vi "信号光谱5.vi"() -> ()   [LabVIEW 2018]
uses:
  <vilib>/Instr/_visa.llb/VISA Configure Serial Port (Instr).vi
  <vilib>/Utility/file.llb/Write Delimited Spreadsheet (DBL).vi
  <vilib>/Analysis/NI_AALBase.lvlib
  <vilib>/ptbypt/NI_PtbyPt.lvlib
panel:
  in  "阈值条件":dbl
  in  "判断角度":dbl
  in  "input parameter":string="D:\\1.jpg"
  out "error out 3":errorcluster
  out "error out 2":errorcluster
  out "照明光":bool
  in  "stop bits (10: 1 bit)":u16(ring)=10 items=["1.0"=10, "1.5"=15, "2.0"=20]
  in  "parity (0:none)":enum16{"None", "Odd", "Even", "Mark", "Space"}(ring)
  in  "data bits (8)":u16=8 min=5 max=8 step=1
  in  "baud rate":u32=9600 caption="baud rate (115200)" min=9600 max=115200
  in  "VISA resource name":refnum<visa-resource-name>="COM3"
  out "正在测量":bool
  in  "滤波阈值":dbl=1500.0 format="%#_13g"
  out "best fit":dbl[][](graph) caption="最佳拟合"
  out "范围内？":bool[](array[boolean])
  out "w":dbl
  out "xc":dbl
  out "拟合参数":dbl[](array[numeric])
  out "最终存储路径":path
  in  "停止程序":bool
  in  "上升下降沿/s":dbl format="%.2p"
  in  "延时/s":dbl format="%.2p"
  in  "占空比/%":dbl=3.0 format="%.2p"
  in  "高电平/V":dbl=4.0 format="%.2p"
  in  "频率/Hz":dbl=100.0 format="%.3p"
  in  "低电平/V":dbl min=0.0 max=5.0 format="%.2p"
  out "configure error out":errorcluster
  in  "设置参数":bool
  out "output control error  4":errorcluster
  in  "低电平持续输出":bool
  in  "Output 1":bool
  out "output control error  5":errorcluster
  in  "测量高电平/V":dbl=4.0
  out "output control error  2":errorcluster
  in  "开始测量":bool
  in  "上升下降沿":i32(ring)=1 items=["上升沿", "下降沿"]
  in  "channel输出口":i32(ring) items=["Channel 1", "Channel 2"]
  in  "输出信号波形":u16(ring) items=["Pulse"]
  out "output control error  3":errorcluster
  out "Output":bool
  in  "VISA 信号发生器":refnum<visa-resource-name>="USB0::0x1AB1::0x0641::DG4E192200870::INSTR"
  out "Spectrum":cluster{"Y":dbl[], "Y":dbl[]}[](graph)
  in  "计数器":dbl=720.0
  out "波长范围":dbl[](array[numeric])
  in  "选项卡控件":enum32{"IHR 550", "CCD"}(tab)
  in  "Move To\nTarget Positions":bool
  out "Current UniqueID":string="Mono4"
  in  "Mono ID":string(combo)="Mono1"
  in  "Connect":bool
  out "Initialized JY":bool=TRUE
  in  "Force\nInitialization":bool
  in  "Target Grating":string(combo)="2"
  out "Current Description":string="1" caption="Description"
  out "Grating Index":i32=1
  out "Current Grating":dbl=1200.0
  out "Units":string="nm"
  out "Current WL":dbl=897.9988
  out "Exit Mirror\nPosition":i32(ring)=2 items=["EntranceMirror", "ExitMirror", "Front", "Side"]
  out "Entrance Mirror\nPosition":i32(ring)=2 items=["EntranceMirror", "ExitMirror", "Front", "Side"]
  out "Units 2":string="mm"
  out "Front Entrance":dbl
  in  "Target WL":dbl=2670.0
  in  "Exit Mirror":u16(ring)=3 caption="Target Position Exit Mirror" items=["Front"=2, "Side"=3]
  in  "Entrance Mirror":u16(ring)=2 caption="Target Position\nEntrance Mirror" items=["Front"=2, "Side"=3]
  in  "Target\nFront Entrance":dbl=1.0
  in  "Commande tab":T1(tab)
  in  "Area Number to Display":i32
  in  "Reformat":bool
  in  "GAIN":u16(ring)=2 caption="Device Name" items=["High Light", "Best Dynamic Range", "High Sensitivity"]
  in  "ADC":u16(ring) caption="Device Name" items=["20 kHz       ", " 1 MHz       ", " 1 MHz Ultra "]
  in  "Number of Areas :":u16=1 min=1 step=1
  in  "Integration time (ms) :":i16=5000
  out "Uniques ID":u16(ring) items=["CCD1", "CCD2"]
  in  "Device Name":u16(ring) items=["Synapse CCD (Lateral)", "Synapse_IGA (Axial)"]
  in  "Signal type :":enum16{"TTL Rising Edge", "TTL Falling Edge"}(ring)=enum."TTL Falling Edge"
  in  "Trigger Type :":u16(ring) items=["On Start"=1, "Per Acquisition"=2]
  in  "trigSigTypeString":string
  in  "trigEventString":string
  in  "Enable InputTriggers :":bool
  in  "Number of Cleans":i32=1
  in  "MultiAcqShutterMode":i32(ring)=3 items=["Open For All Spectra"=1, "Open for Each Spectrum"=3]
  in  "Accumulations:":u16=10 min=1 step=1
  in  "Multi Accumulation mode:":bool
  out "Y Pixels:":i32=256
  out "DataSize":i32=1024
  out "X Pixels:":i32=1024
  out "Firmware\nVersion":string="V1.20 CCD_4000"
  out "initialized ?":bool=TRUE
  in  "Continuous":bool
  in  "CCD Busy":bool
  out "indicator":string="Ready !"
  in  "initialize":bool
  in  "ShutterOpen":bool=TRUE caption="Shutter enable"
  in  "Acquire":bool
  in  "Temperature":bool
  in  "Setup":bool
  in  "起始波长":dbl=2406.79
  in  "终止波长":dbl=2919.91
  out "Acq Time(ms)":u32=3401
  in  "Save Backlight":bool
  in  "cut backlight":bool
  out "backlight":bool=TRUE
  in  "Close":bool=TRUE
  out "JYCCDLib.IJYCCDReqd":refnum<k7>
  out "areas :":i32[][](array[numeric])=[[1], [1], [1], [1024], [256], [1], [256]]
  in  "Constante de condition\n(Voir l'aide contextuelle)":bool
  out "temp graph":dbl(graph)=-134.538067
  out "ADC Number":i32[](array[numeric])=[0, 1, 2, 3, 4]
  out "Gain Number":i32[](array[numeric])=[10, 11, 12, 13, 8, 2]
  out "trigAddress":i32
  out "Data":i32[][](graph)
  out "error out":errorcluster
  out "Gratings":dbl[](array[numeric])=[1200.0, 300.0]
  out "Backlight":i32[][](graph)
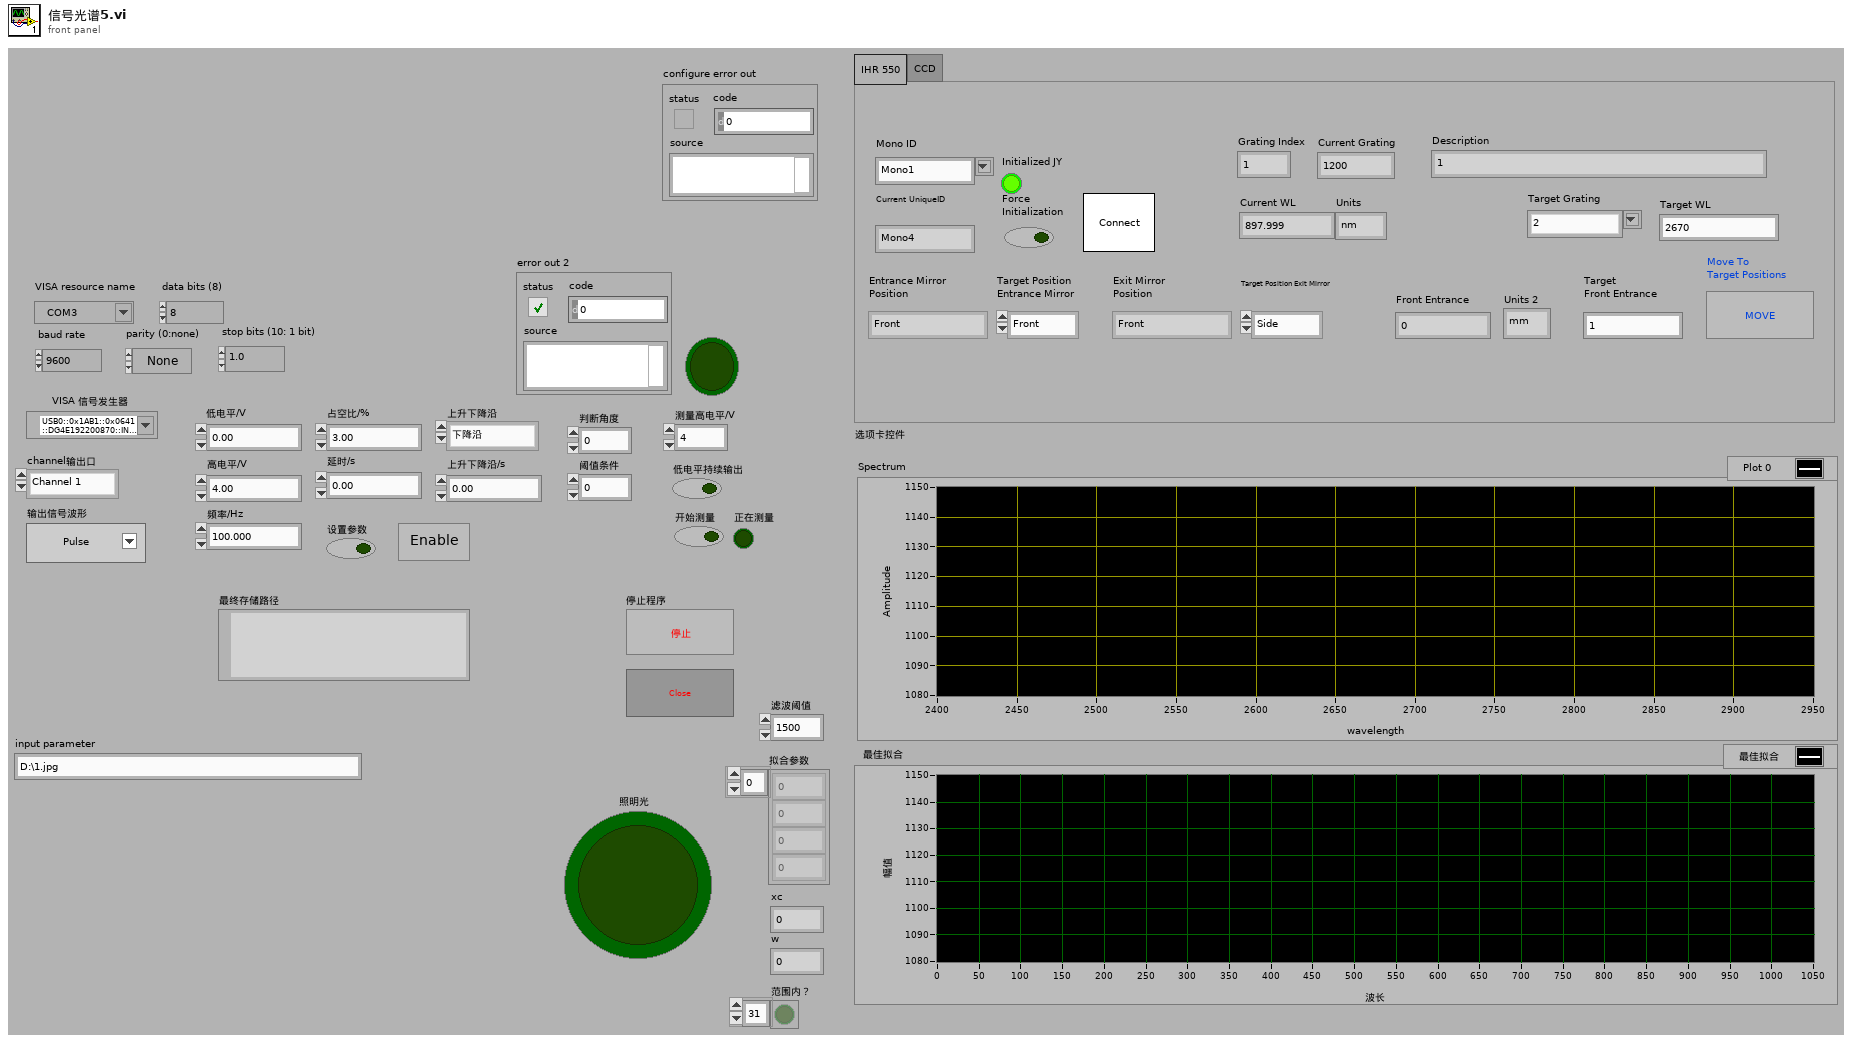
[diagram p1: front panel]
types:
  T1 = enum32{"Settings", "Trigger In", "Multi-Accu.", "Infos"}
  T2 = enum8{"Enabled", "Disabled", "Disabled and Grayed Out"}
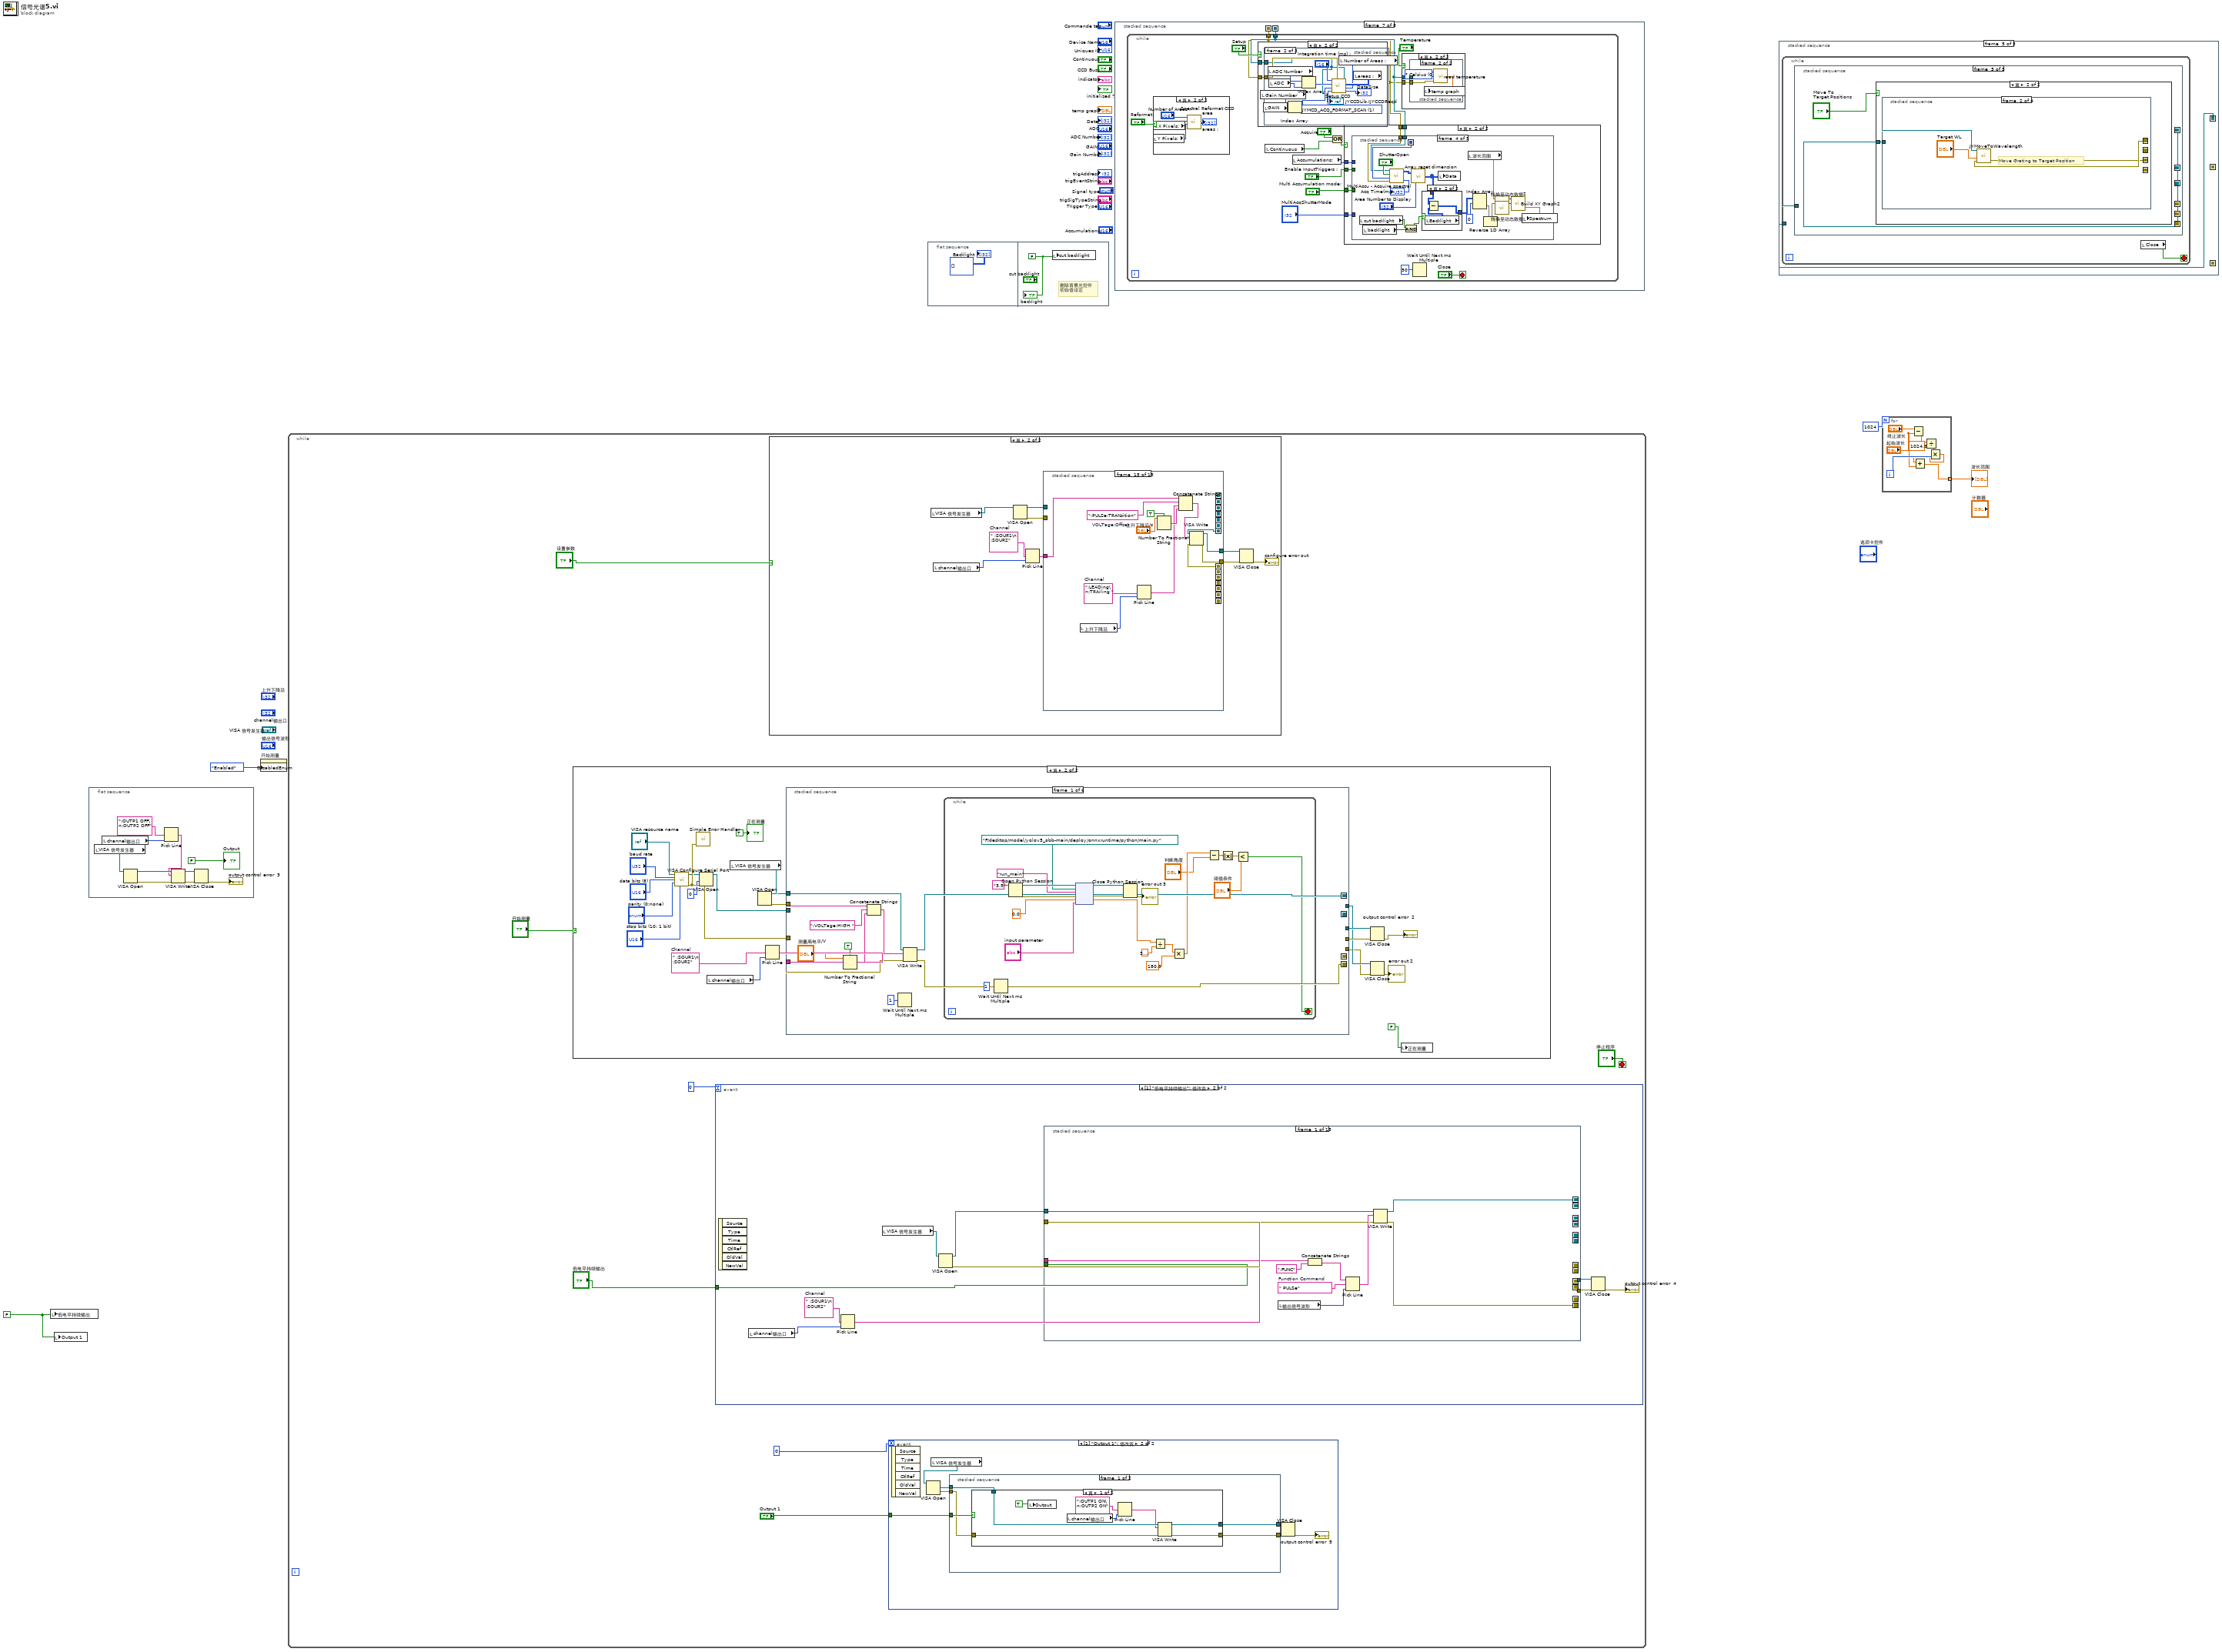
[diagram p0: block diagram]
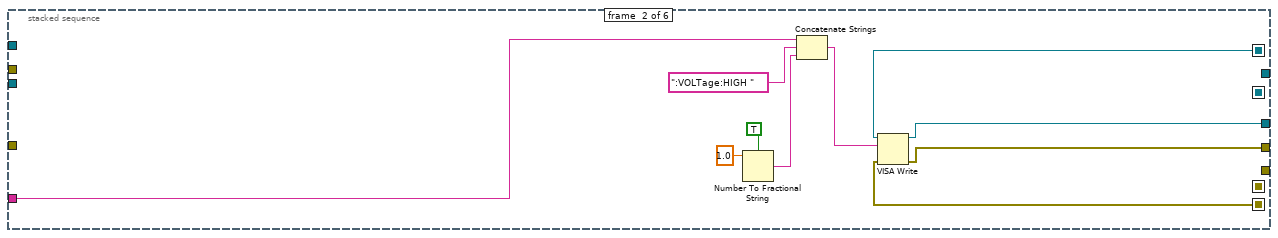
[diagram p3: hidden frame]
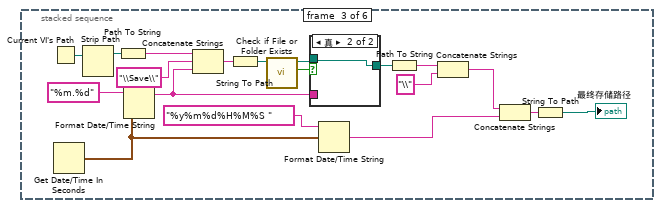
[diagram p4: hidden frame]
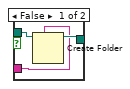
[diagram p5: hidden frame]
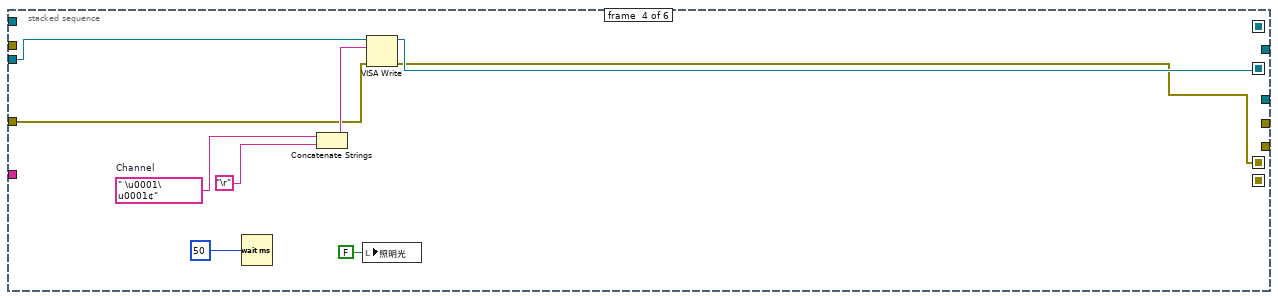
[diagram p6: hidden frame]
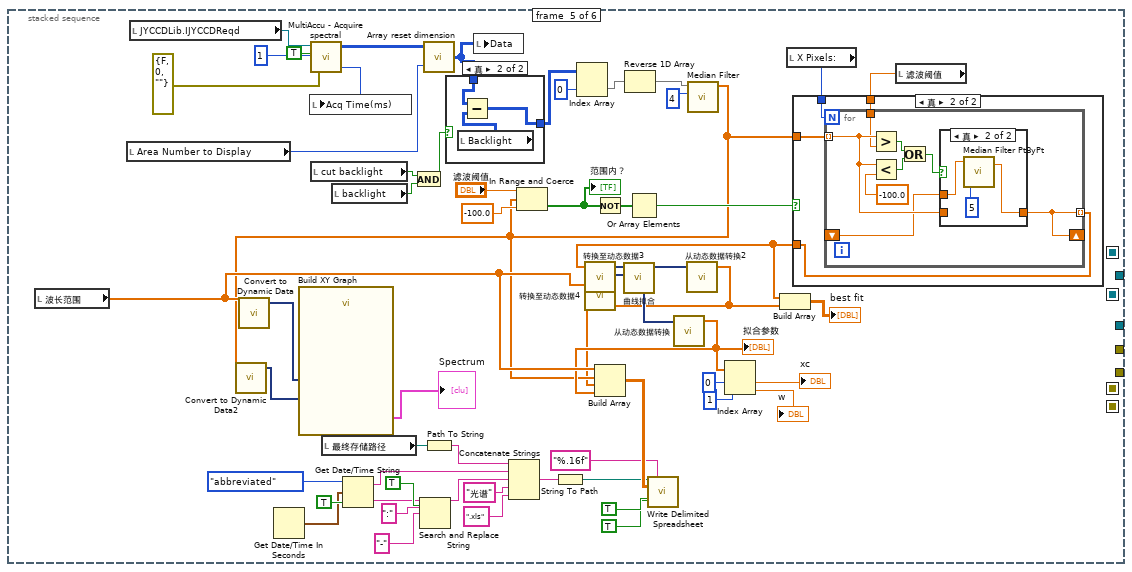
[diagram p7: hidden frame]
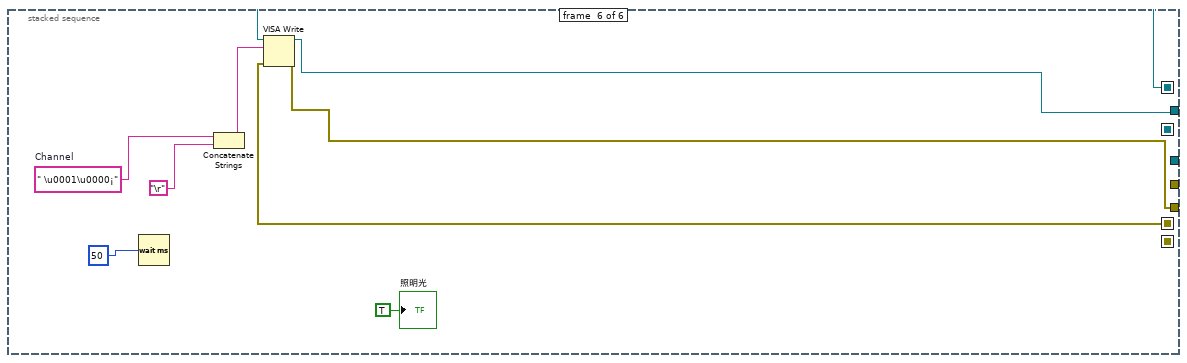
[diagram p11: hidden frame]
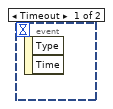
[diagram p12: hidden frame]
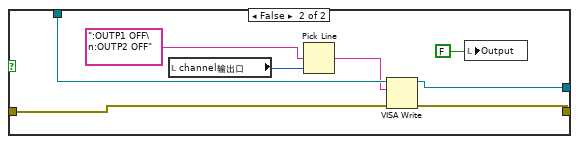
[diagram p13: hidden frame]
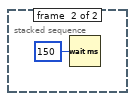
[diagram p14: hidden frame]
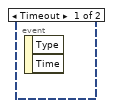
[diagram p15: hidden frame]
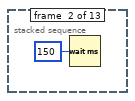
[diagram p16: hidden frame]
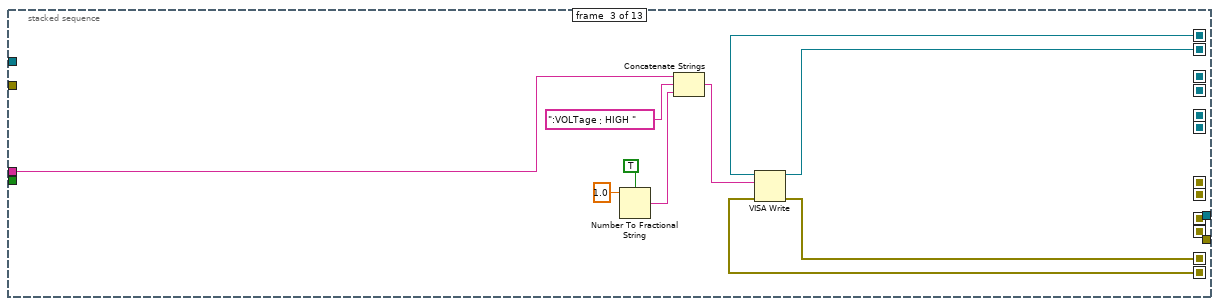
[diagram p17: hidden frame]
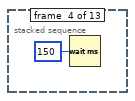
[diagram p18: hidden frame]
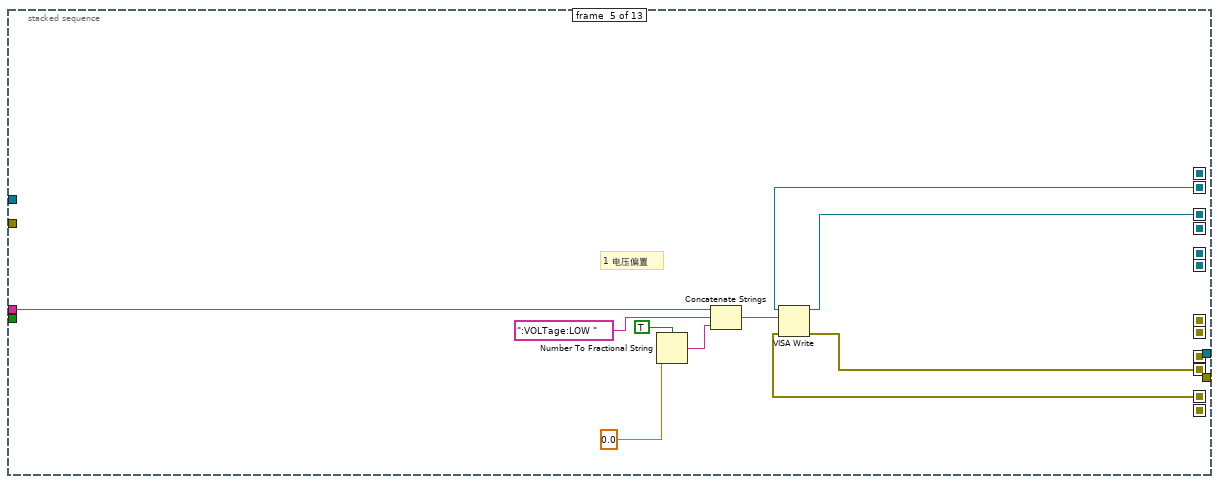
[diagram p19: hidden frame]
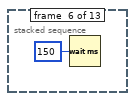
[diagram p20: hidden frame]
diagram:
  w1 = FALSE
  n1 = local write "低电平持续输出"(w1) -> ()
  n2 = local write "Output 1"(w1) -> ()
  n3 = flat-sequence {
    frame #0 {
      n4 = local read "VISA 信号发生器"() -> (w8:refnum<visa-resource-name>)
      n5 = local read "channel输出口"() -> (w6:i32)
      n6 = VISA Open(VISA resource name=w8) -> (VISA resource name=w14:refnum<visa-resource-name>, error out=w13:errorcluster)  [unwired: 4 in]
      n7 = Pick Line(multi-line string=":OUTP1 OFF\n:OUTP2 OFF" ("write buffer"), line index=w6) -> (output string=w5:string)  [unwired: 1 in]
      n8 = VISA Write(VISA resource name=w14, write buffer=w5, error in (no error)=w13) -> (VISA resource name out=w11:refnum<visa-resource-name>, error out=w10:errorcluster)  [unwired: 1 out]
      n9 = VISA Close(VISA resource name=w11, error in (no error)=w10) -> (error out=→"output control error  3":errorcluster)
      "Output" <- FALSE ("布尔")
    }
  }
  n10 = property on="开始测量" class="Bool"("DisabledEnum"=T2."Enabled" ("禁用")) -> ()  [unwired: 2 in, 2 out]
  n11 = while {
    stop <- "停止程序" stop-if-true
    n12 = case shown="真" "开始测量" {
      frame False {
      }
      frame True {
        w37 = " :SOUR1\n :SOUR2"  # Channel
        n13 = call-poly "VISA Configure Serial Port"("VISA resource name"="VISA resource name", "baud rate (9600)"="baud rate", "data bits (8)"="data bits (8)", "parity (0:none)"="parity (0:none)", "stop bits (10: 1 bit)"="stop bits (10: 1 bit)") -> ("VISA resource name out"=w30:refnum<visa-resource-name>, "error out"=w31:errorcluster)  [unwired: 9 in]
        n14 = call <vilib>:"Simple Error Handler.vi"("error in (no error)"=w31) -> ()  [unwired: 4 in, 5 out]
        n15 = VISA Open(access mode=0, error in (no error)=w31, VISA resource name=w30) -> (VISA resource name=w23:refnum<visa-resource-name>, error out=w22:errorcluster)  [unwired: 2 in]
        n16 = local read "channel输出口"() -> (w38:i32)
        n17 = local read "VISA 信号发生器"() -> (w44:refnum<visa-resource-name>)
        n18 = VISA Open(VISA resource name=w44) -> (VISA resource name=w43:refnum<visa-resource-name>, error out=w42:errorcluster)  [unwired: 4 in]
        n19 = Pick Line(multi-line string=w37, line index=w38) -> (output string=w36:string)  [unwired: 1 in]
        n20 = stacked-sequence {
          seq-local: [w48 _ _ _ _ _] -> [_ w80 _ _ _ w202]
          seq-local: [w47 _ _ _ _ _] -> [_ w79 _ _ _ _]
          seq-local: [_ _ _ w112 _ _] -> [_ _ _ _ _ _]
          seq-local: [_ _ _ w111 _ _] -> [_ _ _ _ _ w203]
          tunnel: w43 -> [w51 _ _ _ _ _]
          tunnel: w42 -> [w50 _ _ _ _ _]
          tunnel: [_ w82 _ _ _ _] -> w41
          tunnel: [_ w81 _ _ _ _] -> w40
          tunnel: w36 -> [w52 w78 _ _ _ _]
          tunnel: w23 -> [_ _ _ w115 _ _]
          tunnel: w22 -> [_ _ _ w114 _ _]
          tunnel: [_ _ _ _ _ w201] -> w34
          tunnel: [_ _ _ _ _ w200] -> w33
          frame #0 {
            n21 = Number To Fractional String(use system decimal point (T)=TRUE ("使用系统小数点(T)"), number="测量高电平/V") -> (F-format string=w54:string)  [unwired: 2 in]
            n22 = Concatenate Strings ("连接字符串")(w52, ":VOLTage:HIGH ", w54) -> (w53:string)
            n23 = Wait Until Next ms Multiple(millisecond multiple=u32 1 ("毫秒倍数")) -> ()  [unwired: 1 out]
            n24 = VISA Write(VISA resource name=w51, write buffer=w53, error in (no error)=w50) -> (VISA resource name out=w48:refnum<visa-resource-name>, error out=w47:errorcluster)  [unwired: 1 out]
            n25 = while {
              stop <- w59 stop-if-true
              n26 = Wait Until Next ms Multiple(millisecond multiple=u32 1 ("毫秒倍数")) -> ()  [unwired: 1 out]
              n27 = Open Python Session(python version="3.9" ("Python version")) -> (session out=w76:refnum<k35>, error out=w74:errorcluster)  [unwired: 2 in]
              n28 = node(w76, path "F:/desktop/model/yolov5_obb-main/deploy/onnxruntime/python/main.py" ("module path"), "run_main" ("function name"), w74, 0.0, "input parameter") -> (w75:refnum<k35>, w73:errorcluster, w57:dbl)  [unwired: 1 in, 2 out]
              n29 = Close Python Session(session in=w75, error in=w73) -> (11:→"error out 3":errorcluster)
              n30 = Divide(x=w57, y=3.141592653589793) -> (x/y=w66:dbl)
              n31 = Multiply(x=w66, y=180.0) -> (x*y=w64:dbl)
              n32 = Subtract(x=w64, y="判断角度") -> (x-y=w62:dbl)
              n33 = Absolute Value(x=w62) -> (abs(x)=w61:dbl)
              n34 = Less?(x=w61, y="阈值条件") -> (x < y?=w59:bool)
            }
          }
          frame #1 {
            n35 = Number To Fractional String(use system decimal point (T)=TRUE ("使用系统小数点(T)"), number=1.0 ("数字")) -> (F-format string=w85:string)  [unwired: 2 in]
            n36 = Concatenate Strings ("连接字符串")(w78, ":VOLTage:HIGH ", w85) -> (w84:string)
            n37 = VISA Write(VISA resource name=w80, write buffer=w84, error in (no error)=w79) -> (VISA resource name out=w82:refnum<visa-resource-name>, error out=w81:errorcluster)  [unwired: 1 out]
          }
          frame #2 {
            n38 = Current VI's Path() -> (path=w93:path)
            n39 = Get Date/Time In Seconds() -> (seconds since 1Jan1904=w95:timestamp)
            n40 = Strip Path(path=w93) -> (stripped path=w94:path)  [unwired: 1 out]
            n41 = Path To String(path=w94) -> (string=w96:string)
            n42 = Format Date/Time String(time format string (%c)="%m.%d" ("时间格式字符串(%c)"), seconds (now)=w95) -> (date/time string=w102:string)  [unwired: 1 in]
            n43 = Concatenate Strings(w96, "\\Save\\" ("字符串"), w102) -> (w97:string)
            n44 = String To Path(string=w97) -> (path=w98:path)
            n45 = call <vilib>:"Check if File or Folder Exists.vi"("path"=w98) -> ("file or folder exists?"=w99:bool, "dup path"=w101:path)  [unwired: 8 in, 1 out]
            n46 = case shown="真" w99 {
              tunnel: [w109 w110] -> w100
              tunnel: w101 -> [w108 w110]
              tunnel: w102 -> [w107 _]
              frame False {
                n47 = Create Folder(prompt (Create Folder)=w107, path (use dialog)=w108) -> (created path=w109:path)  [unwired: 1 in, 2 out]
              }
              frame True {
              }
            }
            n48 = Format Date/Time String(time format string (%c)="%y%m%d%H%M%S " ("时间格式字符串(%c)"), seconds (now)=w95) -> (date/time string=w105:string)  [unwired: 1 in]
            n49 = Path To String(path=w100) -> (string=w103:string)
            n50 = Concatenate Strings(w103, "\\" ("字符串")) -> (w104:string)
            n51 = Concatenate Strings(w104, w105) -> (w92:string)
            n52 = String To Path(string=w92) -> (path=→"最终存储路径":path)
          }
          frame #3 {
            w116 = " \u0001\u0001¢"  # Channel
            n53 = Wait (ms)(milliseconds to wait=50) -> ()  [unwired: 1 out]
            n54 = Concatenate Strings(w116, "\r") -> (w117:string)
            n55 = local write "照明光"(FALSE ("照明光")) -> ()
            n56 = VISA Write(VISA resource name=w115, write buffer=w117, error in (no error)=w114) -> (VISA resource name out=w112:refnum<visa-resource-name>, error out=w111:errorcluster)  [unwired: 1 out]
          }
          frame #4 {
            n57 = local read "波长范围"() -> (w142:dbl[])
            n58 = local read "Area Number to Display"() -> (w152:i32)
            n59 = local read "JYCCDLib.IJYCCDReqd"() -> (w148:refnum<k7>)
            n60 = call "Convert to Dynamic Data"("Array"=w142) -> ("Dynamic Data Type"=w145:dynamicdata)  [unwired: 3 in]
            n61 = Get Date/Time In Seconds() -> (seconds since 1Jan1904=w161:timestamp)
            n62 = call "MultiAccu - Acquire spectral.vi"("error in"=errorcluster {"status"=FALSE, "code"=0, "source"=""}, "Accumulations:"=u16 1, "ShutterOpen"=TRUE, "JYCCDLib.IJYCCDReqd"=w148) -> ("Acq Time(ms)"=w154:u32, "Array Out"=w153:i32[][][])  [unwired: 1 out]
            n63 = local write "Acq Time(ms)"(w154) -> ()
            n64 = local read "cut backlight"() -> (w133:bool)
            n65 = local read "最终存储路径"() -> (w175:path)
            n66 = local read "backlight"() -> (w131:bool)
            n67 = Get Date/Time String(date format (0)=enum16{"short", "long", "abbreviated"}."abbreviated" ("日期格式(0)"), seconds (now)=w161, want seconds? (F)=TRUE ("需要秒？(F)")) -> (date string=w169:string, time string=w164:string)
            n68 = And(x=w133, y=w131) -> (x .and. y?=w132:bool)
            n69 = Search and Replace String(replace all?=TRUE ("替换全部？(F)"), input string=w164, search string=":" ("搜索字符串"), replace string="-" ("替换字符串(\"\")")) -> (result string=w168:string)  [unwired: 4 in, 3 out]
            n70 = call "Array reset dimension.vi"("Area Number"=w152, "Array In"=w153) -> ("Array Out"=w135:i32[][])
            n71 = Path To String(path=w175) -> (string=w158:string)
            n72 = case shown="真" w132 {
              tunnel: [w196 w198] -> w134
              tunnel: w135 -> [w196 w197]
              frame False {
              }
              frame True {
                n73 = local read "Backlight"() -> (w199:i32[][])
                n74 = Subtract(x=w197, y=w199) -> (x-y=w198:i32[][])
              }
            }
            n75 = local write "Data"(w135) -> ()
            n76 = Concatenate Strings(w158, w169, w168, "光谱" ("字符串"), ".xls" ("字符串")) -> (w173:string)
            n77 = String To Path(string=w173) -> (path=w174:path)
            n78 = Index Array(array=w134, index (row)=0 ("索引 (行)")) -> (element=w176:i32[])  [unwired: 1 in]
            n79 = call "转换至动态数据4"("Array"=w142) -> ("Dynamic Data Type"=w141:dynamicdata)  [unwired: 3 in]
            n80 = Reverse 1D Array(array=w176) -> (reversed array=w177:i32[])
            n81 = call <vilib>:"Median Filter.vi"("left rank"=4, "X"=w177) -> ("Filtered X"=w126:dbl[])  [unwired: 8 in, 1 out]
            n82 = call "Convert to Dynamic Data2"("Array"=w126) -> ("Dynamic Data Type"=w144:dynamicdata)  [unwired: 3 in]
            n83 = call "Build XY Graph"("Y Input"=w144, "X Input"=w145) -> ("XY Graph"=→"Spectrum":cluster{"Y":dbl[], "Y":dbl[]}[])  [unwired: 8 in, 1 out]
            n84 = In Range and Coerce(upper limit="滤波阈值", x=w126, lower limit=-100.0) -> (In Range?=w125:bool[])  [unwired: 1 out]
            "范围内？" <- w125
            n85 = Not(x=w125) -> (.not. x?=w124:bool[])
            n86 = Or Array Elements(Boolean array=w124) -> (logical OR=w128:bool)
            n87 = local read "X Pixels:"() -> (w127:i32)
            n88 = local read "滤波阈值"() -> (w120:dbl)
            n89 = case shown="真" w128 {
              tunnel: w127 -> [_ w183]
              tunnel: w126 -> [w179 w182]
              tunnel: [w179 w181] -> w123
              tunnel: w120 -> [_ w180]
              frame False {
              }
              frame True {
                n90 = for {
                  N: w183 -> [_]
                  tunnel: w182 -> [w187] mode=indexing
                  tunnel: [w186] -> w181 mode=indexing
                  shift-right: [w186] -> _
                  shift-left: _ -> [w185]
                  tunnel: w180 -> [w184]
                  n91 = Greater?(x=w187, y=w184) -> (0:w189:bool)
                  n92 = Less?(x=w187, y=-100.0) -> (x < y?=w190:bool)
                  n93 = Or(x=w189, y=w190) -> (x .or. y?=w188:bool)
                  n94 = case shown="真" w188 {
                    tunnel: w187 -> [w192 _]
                    tunnel: [w192 w194] -> w186
                    tunnel: w185 -> [_ w195]
                    frame False {
                    }
                    frame True {
                      n95 = call <vilib>:"Median Filter PtByPt.vi"("rank"=5, "x"=w195) -> ("Filtered x"=w194:dbl)  [unwired: 2 in, 1 out]
                    }
                  }
                }
              }
            }
            n96 = call "转换至动态数据3"("Array"=w123) -> ("Dynamic Data Type"=w143:dynamicdata)  [unwired: 3 in]
            n97 = call "曲线拟合"("Locations"=w141, "Signals"=w143) -> ("best fit"=w147:dynamicdata, "non-linear coefficients"=w146:dynamicdata)  [unwired: 5 in, 3 out]
            n98 = call "从动态数据转换"("Dynamic Data Type"=w146) -> ("Array"=w138:dbl[])  [unwired: 3 in]
            "拟合参数" <- w138
            n99 = call "从动态数据转换2"("Dynamic Data Type"=w147) -> ("Array"=w122:dbl[])  [unwired: 3 in]
            n100 = Build Array(w142, w126, w122, w138) -> (w178:dbl[][])
            n101 = call-poly <vilib>:"Write Delimited Spreadsheet.vi"("file path (dialog if empty)"=w174, "format (%.3f)"="%.16f", "2D data"=w178, "append to file? (new file:F)"=TRUE ("append to file? (F)"), "transpose? (no:F)"=TRUE ("transpose? (F)")) -> ()  [unwired: 9 in, 2 out]
            n102 = Index Array(array=w138, index #1=0 ("索引"), index #2=1 ("索引")) -> (element #1=→"xc":dbl, element #2=→"w":dbl)
            n103 = Build Array(w123, w122) -> (→"best fit":dbl[][])
          }
          frame #5 {
            w205 = " \u0001\u0000¡"  # Channel
            n104 = Wait (ms)(milliseconds to wait=50) -> ()  [unwired: 1 out]
            n105 = Concatenate Strings(w205, "\r") -> (w206:string)
            n106 = VISA Write(VISA resource name=w202, write buffer=w206, error in (no error)=w203) -> (VISA resource name out=w201:refnum<visa-resource-name>, error out=w200:errorcluster)  [unwired: 1 out]
            "照明光" <- TRUE ("照明光")
          }
        }
        n107 = VISA Close(VISA resource name=w41, error in (no error)=w40) -> (error out=→"output control error  2":errorcluster)
        n108 = VISA Close(VISA resource name=w34, error in (no error)=w33) -> (error out=→"error out 2":errorcluster)
        n109 = local write "正在测量"(FALSE) -> ()
        "正在测量" <- TRUE
      }
    }
    n110 = event shown="[1] \"低电平持续输出\": 值改变" {
      selector: _ -> [_ _]
      dyn-events: _ -> [_ _]
      timeout: u32 0 ("Time") -> [_ _]
      tunnel: "低电平持续输出" -> [_ w238]
      event Timeout {
        n111 = event-data() -> ()  [unwired: 1 in, 2 out]
      }
      event "低电平持续输出": Value Change {
        w242 = " :SOUR1\n :SOUR2"  # Channel
        n112 = event-data() -> ()  [unwired: 1 in, 6 out]
        n113 = local read "channel输出口"() -> (w243:i32)
        n114 = Pick Line(multi-line string=w242, line index=w243) -> (output string=w241:string)  [unwired: 1 in]
        n115 = local read "VISA 信号发生器"() -> (w246:refnum<visa-resource-name>)
        n116 = VISA Open(VISA resource name=w246) -> (VISA resource name=w245:refnum<visa-resource-name>, error out=w244:errorcluster)  [unwired: 4 in]
        n117 = stacked-sequence {
          seq-local: [w252 _ _ _ _ _ _ _ _ _ _ _ _] -> [_ _ w267 _ _ _ _ _ _ _ _ _ _]
          seq-local: [w251 _ _ _ _ _ _ _ _ _ _ _ _] -> [_ _ w266 _ _ _ _ _ _ _ _ _ _]
          seq-local: [_ _ w265 _ _ _ _ _ _ _ _ _ _] -> [_ _ _ _ w270 _ _ _ _ _ _ _ _]
          seq-local: [_ _ w264 _ _ _ _ _ _ _ _ _ _] -> [_ _ _ _ w271 _ _ _ _ _ _ _ _]
          seq-local: [_ _ _ _ w279 _ _ _ _ _ _ _ _] -> [_ _ _ _ _ _ w290 _ _ _ _ _ _]
          seq-local: [_ _ _ _ w278 _ _ _ _ _ _ _ _] -> [_ _ _ _ _ _ w289 _ _ _ _ _ _]
          seq-local: [_ _ _ _ _ _ w283 _ _ _ _ _ _] -> [_ _ _ _ _ _ _ _ w293 _ _ _ _]
          seq-local: [_ _ _ _ _ _ w282 _ _ _ _ _ _] -> [_ _ _ _ _ _ _ _ w292 _ _ _ _]
          seq-local: [_ _ _ _ _ _ _ _ w296 _ _ _ _] -> [_ _ _ _ _ _ _ _ _ _ w307 _ _]
          seq-local: [_ _ _ _ _ _ _ _ w295 _ _ _ _] -> [_ _ _ _ _ _ _ _ _ _ w306 _ _]
          seq-local: [_ _ _ _ _ _ _ _ _ _ w304 _ _] -> [_ _ _ _ _ _ _ _ _ _ _ _ w321]
          seq-local: [_ _ _ _ _ _ _ _ _ _ w303 _ _] -> [_ _ _ _ _ _ _ _ _ _ _ _ w320]
          tunnel: w245 -> [w257 _ _ _ _ _ _ _ _ _ _ _ _]
          tunnel: w244 -> [w250 _ _ _ _ _ _ _ _ _ _ _ _]
          tunnel: w241 -> [w249 _ w263 _ w276 _ w287 _ w297 _ w310 _ _]
          tunnel: [_ _ _ _ _ _ _ _ _ _ _ _ w319] -> w240
          tunnel: [_ _ _ _ _ _ _ _ _ _ _ _ w317] -> w239
          tunnel: w238 -> [_ _ _ _ _ _ _ _ _ _ _ _ w318]
          frame #0 {
            w254 = " PULSe"  # Function Command
            n118 = local read "输出信号波形"() -> (w248:u16)
            n119 = Concatenate Strings(w249, ":FUNC" ("string (\"\")")) -> (w255:string)
            n120 = Pick Line(string ("")=w255, multi-line string=w254, line index=w248) -> (output string=w253:string)
            n121 = VISA Write(VISA resource name=w257, write buffer=w253, error in (no error)=w250) -> (VISA resource name out=w252:refnum<visa-resource-name>, error out=w251:errorcluster)  [unwired: 1 out]
          }
          frame #1 {
            n122 = Wait (ms)(milliseconds to wait=u32 150) -> ()  [unwired: 1 out]
          }
          frame #2 {
            n123 = Number To Fractional String(use system decimal point (T)=TRUE ("使用系统小数点(T)"), number=1.0 ("数字")) -> (F-format string=w261:string)  [unwired: 2 in]
            n124 = Concatenate Strings ("连接字符串")(w263, ":VOLTage：HIGH ", w261) -> (w260:string)
            n125 = VISA Write(VISA resource name=w267, write buffer=w260, error in (no error)=w266) -> (VISA resource name out=w265:refnum<visa-resource-name>, error out=w264:errorcluster)  [unwired: 1 out]
          }
          frame #3 {
            n126 = Wait (ms)(milliseconds to wait=u32 150) -> ()  [unwired: 1 out]
          }
          frame #4 {
            # "1 电压偏置"
            n127 = Number To Fractional String(use system decimal point (T)=TRUE ("使用系统小数点(T)"), number=0.0 ("数字")) -> (F-format string=w274:string)  [unwired: 2 in]
            n128 = Concatenate Strings(w276, ":VOLTage:LOW ", w274) -> (w275:string)
            n129 = VISA Write(VISA resource name=w270, write buffer=w275, error in (no error)=w271) -> (VISA resource name out=w279:refnum<visa-resource-name>, error out=w278:errorcluster)  [unwired: 1 out]
          }
          frame #5 {
            n130 = Wait (ms)(milliseconds to wait=u32 150) -> ()  [unwired: 1 out]
          }
          frame #6 {
            n131 = local read "channel输出口"() -> (w285:i32)
            n132 = Pick Line(multi-line string=":OUTP1:IMPedance \n:OUTP2:IMPedance " ("write buffer"), line index=w285) -> (output string=w284:string)  [unwired: 1 in]
            n133 = Concatenate Strings ("连接字符串")(w287, w284, "INFINITY") -> (w288:string)
            n134 = VISA Write(VISA resource name=w290, write buffer=w288, error in (no error)=w289) -> (VISA resource name out=w283:refnum<visa-resource-name>, error out=w282:errorcluster)  [unwired: 1 out]
          }
          frame #7 {
            n135 = Wait (ms)(milliseconds to wait=u32 150) -> ()  [unwired: 1 out]
          }
          frame #8 {
            n136 = Number To Fractional String(use system decimal point (T)=TRUE ("使用系统小数点(T)"), number=0.0 ("数字")) -> (F-format string=w300:string)  [unwired: 2 in]
            n137 = Concatenate Strings(w297, ":PULSe:DELay ", w300) -> (w298:string)
            n138 = VISA Write(VISA resource name=w293, write buffer=w298, error in (no error)=w292) -> (VISA resource name out=w296:refnum<visa-resource-name>, error out=w295:errorcluster)  [unwired: 1 out]
          }
          frame #9 {
            n139 = Wait (ms)(milliseconds to wait=u32 150) -> ()  [unwired: 1 out]
          }
          frame #10 {
            w311 = ":LEADing\n:TRAiling "  # Channel
            w315 = ":PULSe:TRANsition"  # VOLTage:Offset
            n140 = local read "上升下降沿"() -> (w312:i32)
            n141 = Pick Line(multi-line string=w311, line index=w312) -> (output string=w308:string)  [unwired: 1 in]
            n142 = Number To Fractional String(use system decimal point (T)=TRUE ("使用系统小数点(T)"), number=0.0 ("数字")) -> (F-format string=w309:string)  [unwired: 2 in]
            n143 = Concatenate Strings(w310, w315, w308, w309) -> (w313:string)
            n144 = VISA Write(VISA resource name=w307, write buffer=w313, error in (no error)=w306) -> (VISA resource name out=w304:refnum<visa-resource-name>, error out=w303:errorcluster)  [unwired: 1 out]
          }
          frame #11 {
            n145 = Wait (ms)(milliseconds to wait=u32 150) -> ()  [unwired: 1 out]
          }
          frame #12 {
            n146 = case shown="假" w318 {
              tunnel: w321 -> [w329 w330]
              tunnel: [w328 w337] -> w317
              tunnel: w320 -> [w327 w335]
              tunnel: [w326 w336] -> w319
              frame True {
                n147 = local write "Output"(TRUE ("布尔")) -> ()
                n148 = local read "channel输出口"() -> (w323:i32)
                n149 = Pick Line(multi-line string=":OUTP1 ON\n:OUTP2 ON" ("write buffer"), line index=w323) -> (output string=w322:string)  [unwired: 1 in]
                n150 = VISA Write(VISA resource name=w329, write buffer=w322, error in (no error)=w327) -> (VISA resource name out=w326:refnum<visa-resource-name>, error out=w328:errorcluster)  [unwired: 1 out]
              }
              frame False {
                n151 = local read "channel输出口"() -> (w332:i32)
                n152 = Pick Line(multi-line string=":OUTP1 OFF\n:OUTP2 OFF" ("write buffer"), line index=w332) -> (output string=w331:string)  [unwired: 1 in]
                n153 = VISA Write(VISA resource name=w330, write buffer=w331, error in (no error)=w335) -> (VISA resource name out=w336:refnum<visa-resource-name>, error out=w337:errorcluster)  [unwired: 1 out]
                n154 = local write "Output"(FALSE ("布尔")) -> ()
              }
            }
          }
        }
        n155 = VISA Close(VISA resource name=w240, error in (no error)=w239) -> (error out=→"output control error  4":errorcluster)
      }
    }
    n156 = case shown="真" "设置参数" {
      frame False {
      }
      frame True {
        w343 = " :SOUR1\n :SOUR2"  # Channel
        n157 = local read "VISA 信号发生器"() -> (w339:refnum<visa-resource-name>)
        n158 = local read "channel输出口"() -> (w338:i32)
        n159 = VISA Open(VISA resource name=w339) -> (VISA resource name=w345:refnum<visa-resource-name>, error out=w346:errorcluster)  [unwired: 4 in]
        n160 = Pick Line(multi-line string=w343, line index=w338) -> (output string=w342:string)  [unwired: 1 in]
        n161 = stacked-sequence {
          seq-local: [w351 _ _ _ _ _ _ _ _ _ _ _ _ _ _] -> [_ _ w366 _ _ _ _ _ _ _ _ _ _ _ _]
          seq-local: [w350 _ _ _ _ _ _ _ _ _ _ _ _ _ _] -> [_ _ w365 _ _ _ _ _ _ _ w404 _ _ _ _]
          seq-local: [_ _ w364 _ _ _ _ _ _ _ _ _ _ _ _] -> [_ _ _ _ w375 _ _ _ _ _ _ _ _ _ _]
          seq-local: [_ _ w363 _ _ _ _ _ _ _ _ _ _ _ _] -> [_ _ _ _ w374 _ _ _ _ _ _ _ _ _ _]
          seq-local: [_ _ _ _ w373 _ _ _ _ _ _ _ _ _ _] -> [_ _ _ _ _ _ w381 _ _ _ _ _ _ _ _]
          seq-local: [_ _ _ _ w370 _ _ _ _ _ _ _ _ _ _] -> [_ _ _ _ _ _ w380 _ _ _ _ _ _ _ _]
          seq-local: [_ _ _ _ _ _ w388 _ _ _ _ _ _ _ _] -> [_ _ _ _ _ _ _ _ w399 _ _ _ _ _ _]
          seq-local: [_ _ _ _ _ _ w387 _ _ _ _ _ _ _ _] -> [_ _ _ _ _ _ _ _ w398 _ _ _ _ _ _]
          seq-local: [_ _ _ _ _ _ _ _ w392 _ _ _ _ _ _] -> [_ _ _ _ _ _ _ _ _ _ w405 _ _ _ _]
          seq-local: [_ _ _ _ _ _ _ _ w391 _ _ _ _ _ _] -> [_ _ _ _ _ _ _ _ _ _ _ _ _ _ _]
          seq-local: [_ _ _ _ _ _ _ _ _ _ w401 _ _ _ _] -> [_ _ _ _ _ _ _ _ _ _ _ _ w415 _ _]
          seq-local: [_ _ _ _ _ _ _ _ _ _ w402 _ _ _ _] -> [_ _ _ _ _ _ _ _ _ _ _ _ w414 _ _]
          seq-local: [_ _ _ _ _ _ _ _ _ _ _ _ w413 _ _] -> [_ _ _ _ _ _ _ _ _ _ _ _ _ _ w426]
          seq-local: [_ _ _ _ _ _ _ _ _ _ _ _ w412 _ _] -> [_ _ _ _ _ _ _ _ _ _ _ _ _ _ w425]
          tunnel: w345 -> [w356 _ _ _ _ _ _ _ _ _ _ _ _ _ _]
          tunnel: w346 -> [w349 _ _ _ _ _ _ _ _ _ _ _ _ _ _]
          tunnel: w342 -> [w348 _ w362 _ w369 _ w385 _ w396 _ w406 _ w416 _ w429]
          tunnel: [_ _ _ _ _ _ _ _ _ _ _ _ _ _ w424] -> w341
          tunnel: [_ _ _ _ _ _ _ _ _ _ _ _ _ _ w423] -> w340
          frame #0 {
            w353 = " PULSe"  # Function Command
            n162 = local read "输出信号波形"() -> (w347:u16)
            n163 = Concatenate Strings(w348, ":FUNC" ("string (\"\")")) -> (w354:string)
            n164 = Pick Line(string ("")=w354, multi-line string=w353, line index=w347) -> (output string=w352:string)
            n165 = VISA Write(VISA resource name=w356, write buffer=w352, error in (no error)=w349) -> (VISA resource name out=w351:refnum<visa-resource-name>, error out=w350:errorcluster)  [unwired: 1 out]
          }
          frame #1 {
            n166 = Wait (ms)(milliseconds to wait=u32 150) -> ()  [unwired: 1 out]
          }
          frame #2 {
            n167 = Number To Fractional String(use system decimal point (T)=TRUE ("使用系统小数点(T)"), number="低电平/V") -> (F-format string=w360:string)  [unwired: 2 in]
            n168 = Concatenate Strings ("连接字符串")(w362, ":VOLTage:LOW ", w360) -> (w359:string)
            n169 = VISA Write(VISA resource name=w366, write buffer=w359, error in (no error)=w365) -> (VISA resource name out=w364:refnum<visa-resource-name>, error out=w363:errorcluster)  [unwired: 1 out]
          }
          frame #3 {
            n170 = Wait (ms)(milliseconds to wait=u32 150) -> ()  [unwired: 1 out]
          }
          frame #4 {
            # "1 频率"
            n171 = Concatenate Strings(w369, ":FREQ ") -> (w376:string)
            n172 = Format Into String ("格式化写入字符串")(initial string=w376, "频率/Hz") -> (resulting string=w377:string)  [unwired: 2 in, 1 out]
            n173 = VISA Write(VISA resource name=w375, write buffer=w377, error in (no error)=w374) -> (VISA resource name out=w373:refnum<visa-resource-name>, error out=w370:errorcluster)  [unwired: 1 out]
          }
          frame #5 {
            n174 = Wait (ms)(milliseconds to wait=u32 150) -> ()  [unwired: 1 out]
          }
          frame #6 {
            n175 = Number To Fractional String(use system decimal point (T)=TRUE ("使用系统小数点(T)"), number="高电平/V") -> (F-format string=w382:string)  [unwired: 2 in]
            n176 = Concatenate Strings(w385, ":VOLTage:HIGH ", w382) -> (w384:string)
            n177 = VISA Write(VISA resource name=w381, write buffer=w384, error in (no error)=w380) -> (VISA resource name out=w388:refnum<visa-resource-name>, error out=w387:errorcluster)  [unwired: 1 out]
          }
          frame #7 {
            n178 = Wait (ms)(milliseconds to wait=u32 150) -> ()  [unwired: 1 out]
          }
          frame #8 {
            n179 = local read "channel输出口"() -> (w394:i32)
            n180 = Pick Line(multi-line string=":OUTP1:IMPedance \n:OUTP2:IMPedance " ("write buffer"), line index=w394) -> (output string=w393:string)  [unwired: 1 in]
            n181 = Concatenate Strings ("连接字符串")(w396, w393, "INFINITY") -> (w397:string)
            n182 = VISA Write(VISA resource name=w399, write buffer=w397, error in (no error)=w398) -> (VISA resource name out=w392:refnum<visa-resource-name>, error out=w391:errorcluster)  [unwired: 1 out]
          }
          frame #9 {
            n183 = Wait (ms)(milliseconds to wait=u32 150) -> ()  [unwired: 1 out]
          }
          frame #10 {
            n184 = Number To Fractional String(use system decimal point (T)=TRUE ("使用系统小数点(T)"), number="占空比/%") -> (F-format string=w408:string)  [unwired: 2 in]
            n185 = Concatenate Strings(w406, ":PULSe:DCYCle ", w408) -> (w403:string)
            n186 = VISA Write(VISA resource name=w405, write buffer=w403, error in (no error)=w404) -> (VISA resource name out=w401:refnum<visa-resource-name>, error out=w402:errorcluster)  [unwired: 1 out]
          }
          frame #11 {
            n187 = Wait (ms)(milliseconds to wait=u32 150) -> ()  [unwired: 1 out]
          }
          frame #12 {
            n188 = Number To Fractional String(use system decimal point (T)=TRUE ("使用系统小数点(T)"), number="延时/s") -> (F-format string=w419:string)  [unwired: 2 in]
            n189 = Concatenate Strings(w416, ":PULSe:DELay ", w419) -> (w417:string)
            n190 = VISA Write(VISA resource name=w415, write buffer=w417, error in (no error)=w414) -> (VISA resource name out=w413:refnum<visa-resource-name>, error out=w412:errorcluster)  [unwired: 1 out]
          }
          frame #13 {
            n191 = Wait (ms)(milliseconds to wait=u32 150) -> ()  [unwired: 1 out]
          }
          frame #14 {
            w430 = ":LEADing\n:TRAiling "  # Channel
            w435 = ":PULSe:TRANsition"  # VOLTage:Offset
            n192 = local read "上升下降沿"() -> (w431:i32)
            n193 = Pick Line(multi-line string=w430, line index=w431) -> (output string=w427:string)  [unwired: 1 in]
            n194 = Number To Fractional String(use system decimal point (T)=TRUE ("使用系统小数点(T)"), number="上升下降沿/s") -> (F-format string=w428:string)  [unwired: 2 in]
            n195 = Concatenate Strings(w429, w435, w427, w428) -> (w432:string)
            n196 = VISA Write(VISA resource name=w426, write buffer=w432, error in (no error)=w425) -> (VISA resource name out=w424:refnum<visa-resource-name>, error out=w423:errorcluster)  [unwired: 1 out]
          }
        }
        n197 = VISA Close(VISA resource name=w341, error in (no error)=w340) -> (error out=→"configure error out":errorcluster)
      }
    }
    n198 = event shown="[1] \"Output 1\": 值改变" {
      selector: _ -> [_ _]
      dyn-events: _ -> [_ _]
      timeout: u32 0 ("Time") -> [_ _]
      tunnel: "Output 1" -> [_ w213]
      event Timeout {
        n199 = event-data() -> ()  [unwired: 1 in, 2 out]
      }
      event "Output 1": Value Change {
        n200 = event-data() -> ()  [unwired: 1 in, 6 out]
        n201 = local read "VISA 信号发生器"() -> (w209:refnum<visa-resource-name>)
        n202 = VISA Open(VISA resource name=w209) -> (VISA resource name=w212:refnum<visa-resource-name>, error out=w215:errorcluster)  [unwired: 4 in]
        n203 = stacked-sequence {
          tunnel: w213 -> [w220 _]
          tunnel: w215 -> [w219 _]
          tunnel: w212 -> [w218 _]
          tunnel: [w217 _] -> w211
          tunnel: [w216 _] -> w210
          frame #0 {
            n204 = case shown="真" w220 {
              tunnel: w218 -> [w228 w236]
              tunnel: [w227 w235] -> w216
              tunnel: w219 -> [w226 w233]
              tunnel: [w225 w234] -> w217
              frame True {
                n205 = local write "Output"(TRUE ("布尔")) -> ()
                n206 = local read "channel输出口"() -> (w222:i32)
                n207 = Pick Line(multi-line string=":OUTP1 ON\n:OUTP2 ON" ("write buffer"), line index=w222) -> (output string=w221:string)  [unwired: 1 in]
                n208 = VISA Write(VISA resource name=w228, write buffer=w221, error in (no error)=w226) -> (VISA resource name out=w225:refnum<visa-resource-name>, error out=w227:errorcluster)  [unwired: 1 out]
              }
              frame False {
                n209 = local read "channel输出口"() -> (w230:i32)
                n210 = Pick Line(multi-line string=":OUTP1 OFF\n:OUTP2 OFF" ("write buffer"), line index=w230) -> (output string=w229:string)  [unwired: 1 in]
                n211 = VISA Write(VISA resource name=w236, write buffer=w229, error in (no error)=w233) -> (VISA resource name out=w234:refnum<visa-resource-name>, error out=w235:errorcluster)  [unwired: 1 out]
                n212 = local write "Output"(FALSE ("布尔")) -> ()
              }
            }
          }
          frame #1 {
            n213 = Wait (ms)(milliseconds to wait=u32 150) -> ()  [unwired: 1 out]
          }
        }
        n214 = VISA Close(VISA resource name=w211, error in (no error)=w210) -> (error out=→"output control error  5":errorcluster)
      }
    }
  }
  n215 = flat-sequence {
    frame #0 {
      "Backlight" <- i32[][] [] ("Backlight")
    }
    frame #1 {
      w437 = FALSE
      # "删除背景光控件\n初始值设定"
      n216 = local write "cut backlight"(w437) -> ()
      "backlight" <- w437
    }
  }
  n217 = stacked-sequence {
    seq-local: [_ _ _ w458 _ _ _ _] -> [_ _ _ _ w476 w496 w499 w604]
    seq-local: [_ _ _ w457 _ _ _ _] -> [_ _ _ _ w477 w497 w498 w605]
    frame #0 {
      # "initialize all variables"
      n218 = property on="initialize" class="Bool"("Désactivé"=u8 0) -> ()  [unwired: 2 in, 2 out]
      n219 = property on="Acquire" class="Bool"("Visible"=FALSE) -> ()  [unwired: 2 in, 2 out]
      n220 = property on="Setup" class="Bool"("Visible"=FALSE) -> ()  [unwired: 2 in, 2 out]
      n221 = local write "indicator"("" ("indicator")) -> ()
      n222 = local write "initialized ?"(FALSE ("initialized ?")) -> ()
      n223 = local write "Continuous"(FALSE ("Continuous")) -> ()
      n224 = local write "Close"(FALSE ("Close")) -> ()
      n225 = property on="Device Name" class="Ring (严格)"("Désactivé"=u8 0) -> ()  [unwired: 2 in, 2 out]
      n226 = property on="Continuous" class="Bool (严格)"("Visible"=FALSE) -> ()  [unwired: 2 in, 2 out]
      n227 = local write "Commande tab"(T1."Settings" ("Commande tab")) -> ()
    }
    frame #1 {
      # "Read Uniq ID"
      n228 = stacked-sequence {
        frame #0 {
          n229 = call "read detector uniq-id.vi"() -> ("nbr of components"=w450:i32, "UniqueID"=w449:string[], "Name"=w448:string[])  [unwired: 4 out]
          n230 = for {
            N: w450 -> [_]
            tunnel: w449 -> [w452]
            tunnel: w448 -> [w451]
            n231 = property on="Device Name" class="Ring (严格)"("Chaînes []"=w451) -> ()  [unwired: 2 in, 2 out]
            n232 = property on="Uniques ID" class="Ring (严格)"("Chaînes []"=w452) -> ()  [unwired: 2 in, 2 out]
          }
        }
      }
    }
    frame #2 {
      n233 = while {
        stop <- "initialize" stop-if-true
        n234 = local read "Device Name"() -> (w455:u16)
        n235 = local write "Uniques ID"(w455) -> ()
        n236 = local read "Close"() -> (w453:bool)
        n237 = Stop(stop? (T)=w453) -> ()
        n238 = Wait Until Next ms Multiple(millisecond multiple=u32 100 ("n millisecondes")) -> ()  [unwired: 1 out]
      }
    }
    frame #3 {
      n239 = stacked-sequence {
        tunnel: [_ w465 _ _] -> w458
        tunnel: [_ w464 _ _] -> w457
        frame #0 {
          n240 = local write "indicator"("Initializing ..." ("indicator")) -> ()
        }
        frame #1 {
          n241 = local read "Uniques ID"() -> (w462:u16)
          n242 = property on="Uniques ID" class="Ring (严格)"() -> ("Chaînes []"=w463:string[])  [unwired: 2 in, 2 out]
          n243 = Index Array(array=w463, index=w462) -> (element=w461:string)
          n244 = call "Initialize CCD.vi"("Unique id:"=w461) -> ("activeYPixels"=→"Y Pixels:":i32, "JYCCDLib.IJYCCDReqd"=w464:refnum<k7>, "activeXPixels"=→"X Pixels:":i32, "sortie d'erreur"=w465:errorcluster, "FirmwareVersion"=→"Firmware\nVersion":string)  [unwired: 3 out]
        }
        frame #2 {
          n245 = property on="initialize" class="Bool"("Désactivé"=u8 2) -> ()  [unwired: 2 in, 2 out]
          n246 = property on="Device Name" class="Ring (严格)"("Désactivé"=u8 2) -> ()  [unwired: 2 in, 2 out]
          n247 = local write "Continuous"(FALSE ("Continuous")) -> ()
          n248 = property on="Setup" class="Bool"("Visible"=TRUE) -> ()  [unwired: 2 in, 2 out]
        }
        frame #3 {
          n249 = local write "initialized ?"(TRUE ("initialized ?")) -> ()
          n250 = local write "indicator"("Initialized !" ("indicator")) -> ()
        }
      }
    }
    frame #4 {
      # "Actually not working"
      # "Read ADC and GAIN"
      n251 = case shown="真" "Constante de condition\n(Voir l'aide contextuelle)" {
        tunnel: w477 -> [_ w487]
        tunnel: w476 -> [_ w486]
        frame False {
        }
        frame True {
          # "Read Input supported trigger"
          n252 = call "Trigger - Get Supported Input.vi"("JYCCDLib.IJYCCDReqd"=w487, "Error Input"=w486) -> ("trigAddress"=w481:i32, "eventPtr"=w482:i32, "trigEventString"=w485:string, "trigSigType"=w484:i32, "trigSigTypeString"=w483:string)  [unwired: 4 out]
          n253 = local write "trigSigTypeString"(w483) -> ()
          n254 = local write "trigAddress"(w481) -> ()
          n255 = local write "Trigger Type :"(w482) -> ()
          n256 = local write "trigEventString"(w485) -> ()
          n257 = local write "Signal type :"(w484) -> ()
        }
      }
      n258 = call "Init ADC & Gain.vi"("JYCCDLib.IJYCCDReqd"=w477, "input error"=w476) -> ("ADC Number"=w475:i32[], "ADC description"=w480:string[], "Gain Number"=w478:i32[], "Gain description"=w479:string[])
      n259 = local write "Gain Number"(w478) -> ()
      n260 = local write "ADC Number"(w475) -> ()
      n261 = stacked-sequence {
        tunnel: w480 -> [w488 _]
        tunnel: w479 -> [_ w489]
        frame #0 {
          n262 = property on="ADC" class="Ring (严格)"("Chaînes []"=w488) -> ()  [unwired: 2 in, 2 out]
        }
        frame #1 {
          n263 = property on="GAIN" class="Ring (严格)"("Chaînes []"=w489) -> ()  [unwired: 2 in, 2 out]
        }
      }
    }
    frame #5 {
      # "IS multi Accumulation Supported ?"
      n264 = call "MultiAccu - Is Supported.vi"("Error In"=w496, "JYCCDLib.IJYCCDReqd"=w497) -> ("IsOperatingModeSupported"=w490:bool)  [unwired: 3 out]
      n265 = Select(t=0, s=w490, f=2) -> (s? t:f=w493:i32)
      n266 = Select(t=FALSE, s=w490, f=w490) -> (s? t:f=w492:bool)
      n267 = local write "Multi Accumulation mode:"(w492) -> ()
      n268 = property on="Multi Accumulation mode:" class="Bool (严格)"("Désactivé"=w493) -> ()  [unwired: 2 in, 2 out]
      n269 = property on="Multi Accumulation mode:" class="Bool (严格)"("Désactivé"=w493) -> ()  [unwired: 2 in, 2 out]
    }
    frame #6 {
      n270 = while {
        tunnel: w498 -> [w506]
        tunnel: w499 -> [w505]
        stop <- "Close" stop-if-true
        n271 = case shown="真" "Reformat" {
          frame False {
          }
          frame True {
            n272 = local read "Y Pixels:"() -> (w582:i32)
            n273 = local read "X Pixels:"() -> (w584:i32)
            n274 = call "Spectral Reformat CCD area.vi"("Y Pixels:"=w582, "X Pixels:"=w584, "numAreas"="Number of Areas :") -> ("areas :"=→"areas :":i32[][])  [unwired: 3 out]
          }
        }
        n275 = case shown="真" "Setup" {
          tunnel: w505 -> [_ w587]
          tunnel: w506 -> [_ w586]
          frame False {
          }
          frame True {
            n276 = stacked-sequence {
              tunnel: w587 -> [_ w601 _]
              tunnel: w586 -> [_ w589 _]
              frame #0 {
                n277 = local write "indicator"("Setting up the detector" ("indicator")) -> ()
              }
              frame #1 {
                w599 = 1 items=["JYMCD_ACQ_FORMAT_IMAGE", "JYMCD_ACQ_FORMAT_SCAN"] ("Acquisition type")
                n278 = local read "Gain Number"() -> (w594:i32[])
                n279 = local read "GAIN"() -> (w590:u16)
                n280 = local read "ADC Number"() -> (w595:i32[])
                n281 = local read "ADC"() -> (w591:u16)
                n282 = Index Array(array=w594, index=w590) -> (element=w592:i32)
                n283 = Index Array(array=w595, index=w591) -> (element=w593:i32)
                n284 = local read "Number of Areas :"() -> (w597:u16)
                n285 = local read "areas :"() -> (w598:i32[][])
                n286 = call "Setup CCD.vi"("numAreas"=w597, "areas :"=w598, "JYCCDLib.IJYCCDReqd"=w589, "entrée d'erreur (pas d'erreur)"=w601, "Acquisition type"=w599, "Gain"=w592, "Select ADC"=w593, "Integration time(ms)"="Integration time (ms) :") -> ("DataSize"=→"DataSize":i32)  [unwired: 1 out]
                "JYCCDLib.IJYCCDReqd" <- w589
              }
              frame #2 {
                w602 = TRUE ("Visible")
                n287 = property on="Continuous" class="Bool (严格)"("Visible"=w602) -> ()  [unwired: 2 in, 2 out]
                n288 = property on="Acquire" class="Bool"("Visible"=w602) -> ()  [unwired: 2 in, 2 out]
                n289 = local write "indicator"("Ready !" ("indicator")) -> ()
              }
            }
          }
        }
        n290 = local read "Continuous"() -> (w507:bool)
        n291 = local read "Accumulations:"() -> (w502:u16)
        n292 = Or(x="Acquire", y=w507) -> (x .or. y?=w504:bool)
        n293 = case shown="真" w504 {
          tunnel: w506 -> [_ w519]
          tunnel: w505 -> [_ w518]
          tunnel: "Enable InputTriggers :" -> [_ w517]
          tunnel: "Multi Accumulation mode:" -> [_ w516]
          tunnel: w502 -> [_ w515]
          tunnel: "MultiAcqShutterMode" -> [_ w514]
          frame False {
          }
          frame True {
            n294 = stacked-sequence {
              seq-local: [_ _ w532 _ _] -> [_ _ _ w562 _]
              tunnel: w519 -> [_ w521 w536 w561 _]
              tunnel: w518 -> [_ w522 w535 w560 _]
              tunnel: w517 -> [_ w523 _ _ _]
              tunnel: w516 -> [_ _ w534 _ _]
              tunnel: w515 -> [_ _ w533 _ _]
              tunnel: w514 -> [_ _ w531 _ _]
              frame #0 {
                n295 = local write "CCD Busy"(TRUE ("CCD Busy")) -> ()
              }
              frame #1 {
                n296 = case shown="真" w523 {
                  tunnel: w522 -> [w524 w530]
                  tunnel: w521 -> [w525 w529]
                  frame False {
                    n297 = call "Trigger - Disable.vi"("Error In"=w524, "JYCCDLib.IJYCCDReqd"=w525) -> ()  [unwired: 6 out]
                  }
                  frame True {
                    n298 = local read "Trigger Type :"() -> (w526:u16)
                    n299 = local read "Signal type :"() -> (w527:enum16{"TTL Rising Edge", "TTL Falling Edge"})
                    n300 = local read "trigAddress"() -> (w528:i32)
                    n301 = call "Trigger - Enable.vi"("Error In"=w530, "sigType"=w527, "event"=w526, "trigAddress"=w528, "JYCCDLib.IJYCCDReqd"=w529) -> ()  [unwired: 3 out]
                  }
                }
              }
              frame #2 {
                n302 = case shown="真" w534 {
                  selector: w534 -> [_ w542]
                  tunnel: w536 -> [w539 w545]
                  tunnel: w535 -> [w538 w544]
                  tunnel: w533 -> [_ w543]
                  tunnel: [u16 1 ("Accumulations:") w543] -> w532
                  tunnel: w531 -> [_ w541]
                  frame False {
                    n303 = call "MultiAccu - Disable.vi"("Error In"=w538, "JYCCDLib.IJYCCDReqd"=w539) -> ()  [unwired: 4 out]
                  }
                  frame True {
                    n304 = call "MultiAccu - Configure.vi"("JYCCDLib.IJYCCDReqd"=w545, "Cleans Before"="Number of Cleans", "Accumulations:"=w543, "MultiAcqHardwareMode"=w542, "MultiAcqShutterMode"=w541, "Error In"=w544) -> ()  [unwired: 1 in, 9 out]
                  }
                }
              }
              frame #3 {
                n305 = local read "cut backlight"() -> (w547:bool)
                n306 = local read "backlight"() -> (w546:bool)
                n307 = call "MultiAccu - Acquire spectral.vi"("error in"=w560, "Accumulations:"=w562, "ShutterOpen"="ShutterOpen", "JYCCDLib.IJYCCDReqd"=w561) -> ("Acq Time(ms)"=→"Acq Time(ms)":u32, "Array Out"=w559:i32[][][])  [unwired: 1 out]
                n308 = And(x=w547, y=w546) -> (x .and. y?=w548:bool)
                n309 = call "Array reset dimension.vi"("Area Number"="Area Number to Display", "Array In"=w559) -> ("Array Out"=w549:i32[][])
                n310 = case shown="真" w548 {
                  tunnel: [w565 w566] -> w550
                  tunnel: w549 -> [w565 w567]
                  frame False {
                  }
                  frame True {
                    n311 = local read "Backlight"() -> (w568:i32[][])
                    n312 = Subtract(x=w567, y=w568) -> (x-y=w566:i32[][])
                  }
                }
                n313 = local write "Data"(w549) -> ()
                n314 = local read "波长范围"() -> (w553:dbl[])
                n315 = Index Array(array=w550, index (row)=0 ("禁用的索引 (列)")) -> (element=w552:i32[])  [unwired: 1 in]
                n316 = Reverse 1D Array(array=w552) -> (reversed array=w551:i32[])
                n317 = call "转换至动态数据2"("Array"=w553) -> ("Dynamic Data Type"=w555:dynamicdata)  [unwired: 3 in]
                n318 = call "转换至动态数据"("Array"=w551) -> ("Dynamic Data Type"=w556:dynamicdata)  [unwired: 3 in]
                n319 = call "Build XY Graph2"("Y Input"=w556, "X Input"=w555) -> ("XY Graph"=w554:cluster{"Y":dbl[], "Y":dbl[]}[])  [unwired: 8 in, 1 out]
                n320 = local write "Spectrum"(w554) -> ()
              }
              frame #4 {
                n321 = case shown="真" "Save Backlight" {
                  frame False {
                  }
                  frame True {
                    w571 = TRUE ("删除背景光")
                    n322 = local read "Data"() -> (w573:i32[][])
                    n323 = local write "Backlight"(w573) -> ()
                    n324 = local write "cut backlight"(w571) -> ()
                    n325 = local write "backlight"(w571) -> ()
                    n326 = local write "Save Backlight"(FALSE ("Save Backlight")) -> ()
                  }
                }
                n327 = local write "CCD Busy"(FALSE ("CCD Busy")) -> ()
              }
            }
          }
        }
        n328 = case shown="真" "Temperature" {
          tunnel: w506 -> [_ w576]
          tunnel: w505 -> [_ w575]
          frame False {
            n329 = property on="temp graph" class="WFChart (严格)"("Visible"=FALSE) -> ()  [unwired: 2 in, 2 out]
          }
          frame True {
            n330 = stacked-sequence {
              tunnel: w576 -> [_ w581]
              tunnel: w575 -> [_ w580]
              frame #0 {
                n331 = property on="temp graph" class="WFChart (严格)"("Visible"=TRUE) -> ()  [unwired: 2 in, 2 out]
              }
              frame #1 {
                w579 = u16 0 items=["° Celsius", "Kelvin", "° Farenheit"] ("units")
                n332 = call "read temperature.vi"("entrée d'erreur (pas d'erreur)"=w580, "units"=w579, "JYCCDLib.IJYCCDReqd"=w581) -> ("Current Temperature"=w578:dbl)
                n333 = local write "temp graph"(w578) -> ()
              }
            }
          }
        }
        n334 = Wait Until Next ms Multiple(millisecond multiple=u32 50 ("n millisecondes")) -> ()  [unwired: 1 out]
      }
    }
    frame #7 {
      n335 = Close Reference(reference=w605, error in (no error)=w604) -> ()  [unwired: 1 out]
    }
  }
  n336 = stacked-sequence {
    seq-local: [_ _ w615 _ _] -> [_ _ _ w625 w630]
    seq-local: [_ _ w614 _ _] -> [_ _ _ w624 _]
    seq-local: [_ _ _ w623 _] -> [_ _ _ _ _]
    frame #0 {
      n337 = call "Get Monos From Config Browser.vi"() -> ("UniqueIDs"=w610:string[], "Mono ID"=w611:string[])  [unwired: 3 in, 1 out]
      n338 = Build Cluster Array(w611, w610) -> (w608:cluster{"String":string, "String":string}[])
      n339 = property on="Mono ID" class="CmbBox"("Strings And Values []"=w608) -> ()  [unwired: 2 in, 2 out]
      n340 = Index Array(array=w608, index=0) -> (element=w609:cluster{"String":string, "String":string})
      n341 = Unbundle(w609) -> ("String"=w606:string)  [unwired: 1 out]
      "Current UniqueID" <- w606
      n342 = local write "Mono ID"(w606) -> ()
    }
    frame #1 {
      n343 = while {
        stop <- "Connect" stop-if-true
        n344 = local read "Mono ID"() -> (w612:string)
        n345 = local write "Current UniqueID"(w612) -> ()
      }
    }
    frame #2 {
      n346 = local read "Mono ID"() -> (w617:string)
      n347 = call "JYInitMono.vi"("Unique ID"=w617, "Force Init"="Force\nInitialization") -> ("Refnum out"=w615:refnum<k7>, "Initialized"=→"Initialized JY":bool, "error out"=w614:errorcluster)  [unwired: 9 in, 2 out]
    }
    frame #3 {
      n348 = call "Show Current Grating.vi"("Refnum in"=w625, "error in (no error)"=w624) -> ("Gratings"=w626:dbl[], "Grating Index"=w620:i32, "Current Grating"=w622:dbl, "Current Description"=w619:string, "error out"=w623:errorcluster)  [unwired: 5 in, 4 out]
      "Gratings" <- w626
      n349 = local write "Current Grating"(w622) -> ()
      n350 = local write "Current Description"(w619) -> ()
      n351 = Number To Decimal String(number=w626) -> (decimal integer string=w628:string[])  [unwired: 1 in]
      n352 = Number To Decimal String(number=w620) -> (decimal integer string=w621:string)  [unwired: 1 in]
      n353 = property on="Target Grating" class="CmbBox"("Value"=w621) -> ()  [unwired: 2 in, 2 out]
      n354 = Build Cluster Array(w628, string[] ["1", "2", "3"]) -> (w629:cluster{"Numeric":string, string}[])
      n355 = property on="Target Grating" class="CmbBox"("Strings And Values []"=w629) -> ()  [unwired: 2 in, 2 out]
    }
    frame #4 {
      n356 = while {
        tunnel: w630 -> [w632]
        stop <- w631 stop-if-true
        n357 = stacked-sequence {
          seq-local: [w636 _ _ _ _] -> [_ w643 w654 _ w662]
          seq-local: [w635 _ _ _ _] -> [_ w642 w653 _ _]
          seq-local: [_ w641 _ _ _] -> [_ _ _ _ _]
          seq-local: [_ w640 _ _ _] -> [_ _ _ _ _]
          seq-local: [_ _ w646 _ _] -> [_ _ _ _ _]
          seq-local: [_ _ w645 _ _] -> [_ _ _ w656 _]
          tunnel: w632 -> [w634 _ _ w657 _]
          frame #0 {
            n358 = call "Show Current Grating.vi"("Refnum in"=w634) -> ("Grating Index"=→"Grating Index":i32, "Current Grating"=→"Current Grating":dbl, "Current Description"=→"Current Description":string, "error out"=w635:errorcluster, "JYMONOLib.IJYMonoReqd"=w636:refnum<k7>)  [unwired: 6 in, 4 out]
          }
          frame #1 {
            n359 = call "JYGetCurrentWL.vi"("error in (no error)"=w642, "JYMONOLib.IJYMonoReqd"=w643) -> ("error out"=w640:errorcluster, "Units"=→"Units":string, "Current WL"=→"Current WL":dbl, "JYMONOLib.IJYMonoReqd 2"=w641:refnum<k7>)  [unwired: 6 in]
          }
          frame #2 {
            w651 = u16 1 items=["Entrance", "Exit"] ("Mirror Number")
            w652 = u16 0 items=["Entrance", "Exit"] ("Mirror Number")
            n360 = call "JYGetMirrorPos.vi"("error in (no error)"=w653, "Mirror"=w652, "Refnum In"=w654) -> ("error out"=w649:errorcluster, "Current Mirror Position"=→"Entrance Mirror\nPosition":i32, "Refnum Out"=w650:refnum<k7>)  [unwired: 1 in]
            n361 = call "JYGetMirrorPos.vi"("error in (no error)"=w649, "Mirror"=w651, "Refnum In"=w650) -> ("error out"=w645:errorcluster, "Current Mirror Position"=→"Exit Mirror\nPosition":i32, "Refnum Out"=w646:refnum<k7>)  [unwired: 1 in]
          }
          frame #3 {
            w659 = u16 0 items=["Front Entrance", "Side Entrance", "Front Exit", "Side Exit", "First Intermediate", "Second Intermediate"] ("Slit")
            n362 = call "JYGetSlits.vi"("MonoRefNum IN"=w657, "Slit"=w659, "error in (no error)"=w656) -> ("Units"=→"Units 2":string, "Slit Width"=→"Front Entrance":dbl, "error out"=→"error out":errorcluster)  [unwired: 13 in, 1 out]
          }
          frame #4 {
            n363 = case shown="真" "Move To\nTarget Positions" {
              tunnel: w662 -> [_ w663]
              frame False {
              }
              frame True {
                n364 = stacked-sequence {
                  seq-local: [w665 _ _ _] -> [_ w671 _ _]
                  seq-local: [_ w669 _ _] -> [_ _ w686 _]
                  seq-local: [_ _ w673 _] -> [_ _ _ w692]
                  seq-local: [_ _ _ w689] -> [_ _ _ _]
                  tunnel: w663 -> [w667 w670 w684 w693]
                  frame #0 {
                    n365 = property on="Target Grating" class="CmbBox"() -> ("Value"=w664:string)  [unwired: 2 in, 2 out]
                    n366 = local read "error out"() -> (w666:errorcluster)
                    n367 = Decimal String To Number(string=w664) -> (number=w668:i32)  [unwired: 2 in, 1 out]
                    n368 = call "JYTurret.vi"("error in (no error)"=w666, "Grating Index"=w668, "JYMONOLib.IJYMonoReqd"=w667) -> ("error out"=w665:errorcluster)  [unwired: 2 out]
                  }
                  frame #1 {
                    # "Move Grating to Target Position"
                    n369 = call "JYMoveToWavelength.vi"("error in (no error)"=w671, "Target WL"="Target WL", "RefNum In"=w670) -> ("error out"=w669:errorcluster)  [unwired: 1 in, 2 out]
                  }
                  frame #2 {
                    w679 = u16 1 items=["Entrance", "Exit"] ("Mirror Number")
                    w678 = u16 0 items=["Entrance", "Exit"] ("Mirror Number")
                    w685 = u16 1 items=["Entrance", "Exit", "Front", "Side"] ("Mirror Number")
                    w688 = u16 0 items=["Entrance", "Exit", "Front", "Side"] ("Mirror Number")
                    # "Move Mirrors"
                    n370 = call "JYMirrorMove.vi"("error in (no error)"=w686, "Mirror Position"="Entrance Mirror", "Mirror Number"=w688, "RefNum In"=w684) -> ("error out"=w683:errorcluster)  [unwired: 6 in, 1 out]
                    n371 = call "JYMirrorMove.vi"("error in (no error)"=w683, "Mirror Position"="Exit Mirror", "Mirror Number"=w685, "RefNum In"=w684) -> ("error out"=w676:errorcluster, "MonoRefNum Out"=w677:refnum<k7>)  [unwired: 6 in]
                    n372 = call "JYGetMirrorPos.vi"("error in (no error)"=w676, "Mirror"=w678, "Refnum In"=w677) -> ("error out"=w681:errorcluster, "Current Mirror Position"=w675:i32, "Refnum Out"=w680:refnum<k7>)  [unwired: 1 in]
                    n373 = local write "Entrance Mirror\nPosition"(w675) -> ()
                    n374 = call "JYGetMirrorPos.vi"("error in (no error)"=w681, "Mirror"=w679, "Refnum In"=w680) -> ("error out"=w673:errorcluster, "Current Mirror Position"=w674:i32)  [unwired: 1 in, 1 out]
                    n375 = local write "Exit Mirror\nPosition"(w674) -> ()
                  }
                  frame #3 {
                    w691 = u16 0 items=["Front Entrance", "Side Entrance", "Front Exit", "Side Exit", "First Intermediate", "Second Intermediate"] ("Slit")
                    # "Set New Slit Positions"
                    n376 = call "JYSlits.vi"("JYMONOLib.IJYMonoReqd"=w693, "Slit"=w691, "error in (no error)"=w692, "Slit Width"="Target\nFront Entrance") -> ("error out"=w689:errorcluster)  [unwired: 1 in, 1 out]
                  }
                }
              }
            }
          }
        }
        n377 = local read "Close"() -> (w631:bool)
      }
    }
  }
  n378 = for {
    N: 1024 -> [_]
    tunnel: [w698] -> w3 mode=indexing
    i -> [w700]
    n379 = Subtract(x="终止波长", y="起始波长") -> (x-y=w696:dbl)
    n380 = Divide(x=w696, y=1024.0) -> (x/y=w694:dbl)
    n381 = Multiply(x=w694, y=w700) -> (x*y=w699:dbl)
    n382 = Add(x=w699, y="起始波长") -> (x+y=w698:dbl)
  }
  "波长范围" <- w3
